vi "squre.vi"(1 "time":dbl, 2 "f":dbl, 3 "Amp":dbl) -> (0 "squre":dbl)   [LabVIEW 2011]
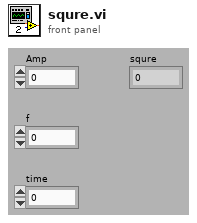
[diagram p1: front panel]
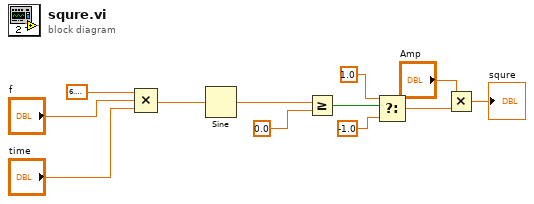
[diagram p0: block diagram]
diagram:
  n1 = Compound Arithmetic op=MULTIPLY(6.283185307179586, "f", "time") -> (w1:dbl)
  n2 = Sine(x=w1) -> (sin(x)=w3:dbl)
  n3 = Greater Or Equal?(x=w3, y=0.0) -> (x >= y?=w5:bool)
  n4 = Select(t=1.0, s=w5, f=-1.0) -> (s? t:f=w10:dbl)
  n5 = Multiply(x="Amp", y=w10) -> (x*y=→"squre":dbl)
